vi "DestroyPrivateEvents.vi"(8 "error in (no error)":errorcluster, 11 "Generator":refnum<class "Generator.lvclass">) -> (0 "error out":errorcluster, 3 "Generator out":refnum<class "Generator.lvclass">)   [LabVIEW 2019, in "Generator.lvclass"]
uses:
  Generator.lvclass
  <vilib>/JKI/JKI SMO/SMO/SMO.lvclass
panel:
  # "For instructions on how to use the JKI State Machine Objects, examples and video tutorials, visit:\nhttp://jki.net/state-machine-objects/\n\nJKI State Machine Objects™\nhttp://jki.net/state-machine-objects/\nCopyright (C) 2005-2015, JKI <info@jki.net>\nALL RIGHTS RESERVED"
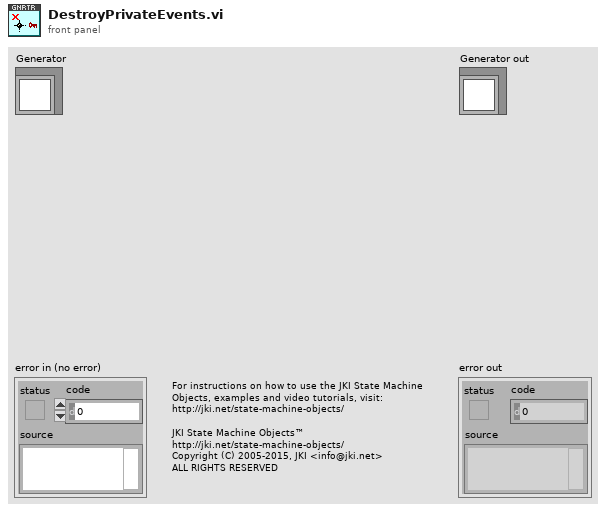
[diagram p1: front panel]
types:
  T1 = typedef "Generator.lvclass/PrivateEvents--Cluster.ctl" = cluster{"Message":refnum<user-event>, "Sampling":refnum<user-event>, "AOchannel":refnum<user-event>, "REFchannel":refnum<user-event>, "Sweep":refnum<user-event>}
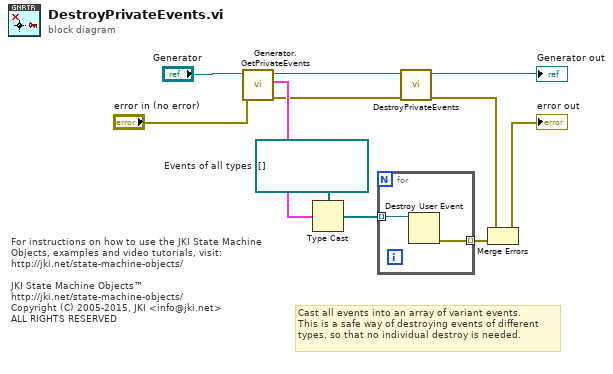
[diagram p0: block diagram]
diagram:
  w9 = refnum<user-event>[] []  # Events of all types
  # "For instructions on how to use the JKI State Machine Objects, examples and video tutorials, visit:\nhttp://jki.net/state-machine-objects/\n\nJKI State Machine Objects™\nhttp://jki.net/state-machine-objects/\nCopyright (C) 2005-2015, JKI <info@jki.net>\nALL RIGHTS RESERVED"
  # "Cast all events into an array of variant events.\nThis is a safe way of destroying events of different\ntypes, so that no individual destroy is needed."
  n1 = call "Generator.GetPrivateEvents.vi"("error in (no error)"="error in (no error)", "Generator"="Generator") -> ("error out"=w2:errorcluster, "Generator Private Events"=w5:T1, "Generator out"=w3:refnum<class "Generator.lvclass">)  [unwired: 7 in]
  n2 = Type Cast(type=w9, x=w5) -> (*(type *) &x=w10:refnum<user-event>[])
  n3 = for {
    tunnel: w10 -> [w13] mode=indexing
    tunnel: [w12] -> w8 mode=indexing
    n4 = Destroy User Event(user event=w13) -> (error out=w12:errorcluster)  [unwired: 1 in]
  }
  n5 = call-parent "DestroyPrivateEvents.vi"("error in (no error)"=w2, "SMO"=w3) -> ("error out"=w11:errorcluster, "SMO out"=→"Generator out":refnum<class "Generator.lvclass">)  [unwired: 8 in]
  n6 = Merge Errors(w11, w8) -> (→"error out":errorcluster)
